vi "DataDecodificator.vi"(8 "?":errorcluster, 10 "Separation Character":string, 11 "Read Buffer":string) -> (0 "error out":errorcluster, 1 "Bearing Accel 3":dbl, 2 "Bearing Accel 2":dbl, 3 "Motor Accel 1":dbl, 4 "Load Accel 4":dbl)   [LabVIEW 2017]
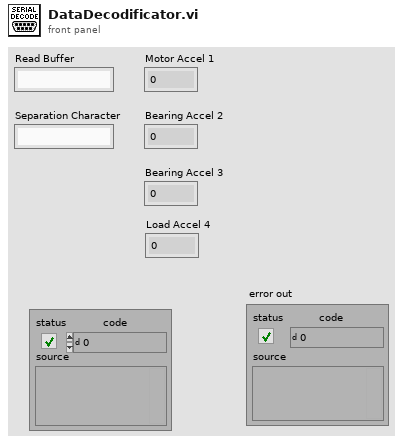
[diagram p1: front panel]
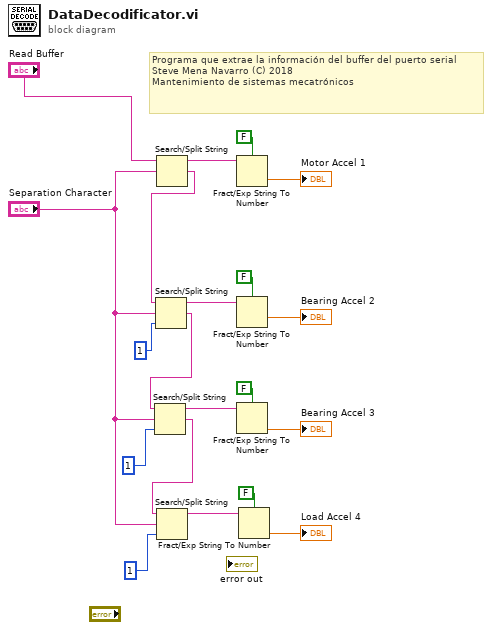
[diagram p0: block diagram]
diagram:
  # "Programa que extrae la información del buffer del puerto serial\nSteve Mena Navarro (C) 2018\nMantenimiento de sistemas mecatrónicos"
  n1 = Search/Split String(string="Read Buffer", search string/char (-)="Separation Character") -> (substring before match=w13:string, match + rest of string=w14:string)  [unwired: 1 in, 1 out]
  n2 = Search/Split String(string=w14, search string/char (-)="Separation Character", offset (0)=1) -> (substring before match=w9:string, match + rest of string=w17:string)  [unwired: 1 out]
  n3 = Search/Split String(string=w17, search string/char (-)="Separation Character", offset (0)=1) -> (substring before match=w10:string, match + rest of string=w2:string)  [unwired: 1 out]
  n4 = Search/Split String(string=w2, search string/char (-)="Separation Character", offset (0)=1) -> (substring before match=w4:string)  [unwired: 2 out]
  n5 = Fract/Exp String To Number(use system decimal point (T)=FALSE, string=w13) -> (number=→"Motor Accel 1":dbl)  [unwired: 2 in, 1 out]
  n6 = Fract/Exp String To Number(use system decimal point (T)=FALSE, string=w9) -> (number=→"Bearing Accel 2":dbl)  [unwired: 2 in, 1 out]
  n7 = Fract/Exp String To Number(use system decimal point (T)=FALSE, string=w10) -> (number=→"Bearing Accel 3":dbl)  [unwired: 2 in, 1 out]
  n8 = Fract/Exp String To Number(use system decimal point (T)=FALSE, string=w4) -> (number=→"Load Accel 4":dbl)  [unwired: 2 in, 1 out]
